vi "Ctor.vi"(8 "error in (no error)":errorcluster, 11 "DeviceArrayPanel in":refnum<class "DeviceArrayPanel.lvclass">) -> (0 "error out":errorcluster, 3 "DeviceArrayPanel out":refnum<class "DeviceArrayPanel.lvclass">)   [LabVIEW 2020, in "PicoG-App.lvlib" / "DeviceArrayPanel.lvclass"]
uses:
  DeviceArrayPanel.lvclass
  Ref Data.ctl
  Device/Device.lvclass
  DeviceArrayPanel.lvclass/DeviceArrayPanel.ctl
  <vilib>/IlluminatedG/IG OOPanel/OOPanel/ArrayPanel/ArrayPanel.lvclass
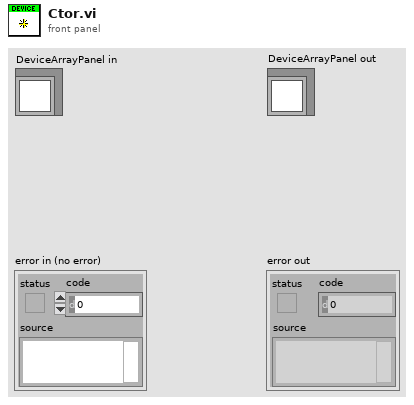
[diagram p1: front panel]
types:
  T1 = typedef "PicoG-App.lvlib/DeviceArrayPanel.lvclass/Ref Data.ctl" = cluster{"Device":refnum<class "Device.lvclass">}
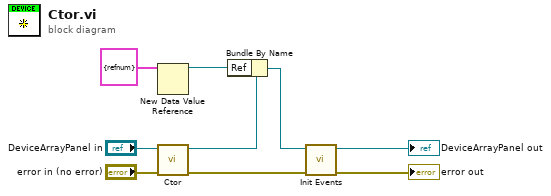
[diagram p0: block diagram]
diagram:
  n1 = New Data Value Reference(data value=T1 {"Device"=refnum} ("Ref Data")) -> (data value reference=w5:refnum<data-value>)  [unwired: 1 in, 1 out]
  n2 = call-parent "Ctor.vi"("error in (no error)"="error in (no error)", "ArrayPanel in"="DeviceArrayPanel in") -> ("error out"=w4:errorcluster, "ArrayPanel out"=w7:refnum<class "DeviceArrayPanel.lvclass">)  [unwired: 8 in]
  n3 = Bundle By Name(cluster=w7, "Ref"=w5) -> (w3:refnum<class "DeviceArrayPanel.lvclass">)
  n4 = call "Init Events.vi"("error in (no error)"=w4, "DeviceArrayPanel in"=w3) -> ("error out"=→"error out":errorcluster, "DeviceArrayPanel out"=→"DeviceArrayPanel out":refnum<class "DeviceArrayPanel.lvclass">)  [unwired: 8 in]
